vi "Actor Core.vi"(8 "error in":errorcluster caption="错误输入", 11 "Programmatic Controller in":refnum<class "Programmatic Controller.lvclass"> caption="操作者输入") -> (0 "error out":errorcluster caption="错误输出", 3 "Actor out":refnum<class "Actor.lvclass"> caption="操作者输出")   [LabVIEW 2017, in "Programmatic Controller.lvclass"]
doc: "(<B>Filename</B>: Actor Framework.lvlib:Actor.lvclass:Actor Core.vi)\n\nReceives messages to the actor, reacts to them, and initiates any error handling that may shut the actor down.\n\nDescendant classes may override this VI to append parallel tasks for the actor to complete while it handles messages. Overrides use the Call Parent Method node."
uses:
  Programmatic Controller.lvclass
  E:/Program Files (x86)/National Instruments/LabVIEW 2017/vi.lib/ActorFramework/Actor/Actor.lvclass
  <vilib>/ActorFramework/Actor/Actor.lvclass
  <vilib>/ActorFramework/Actor/Actor.lvclass/Actor.ctl
  <vilib>/ActorFramework/Message Enqueuer/Message Enqueuer.lvclass/Message Enqueuer.ctl
  <vilib>/Utility/error.llb/DialogType.ctl
  <vilib>/DAQmx/write.llb/DAQmx Write (Digital Bool 1Line 1Point).vi
  <vilib>/DAQmx/write.llb/DAQmx Write (Analog 1D DBL NChan 1Samp).vi
  <vilib>/ActorFramework/Message Enqueuer/Init from Existing Queue.vi
  <vilib>/ActorFramework/Message Enqueuer/Enqueue.vi
  <vilib>/ActorFramework/Stop Msg/Stop Msg.lvclass
  E:/Program Files (x86)/National Instruments/LabVIEW 2017/vi.lib/ActorFramework/Message/Message.lvclass
  <vilib>/ActorFramework/Message Priority Queue/Priority Enqueue.vi
  <vilib>/Utility/file.llb/Read Delimited Spreadsheet (DBL).vi
  <vilib>/DAQmx/create/channels.llb/DAQmx Create Channel (DO-Digital Output).vi
  <vilib>/DAQmx/create/channels.llb/DAQmx Create Channel (AO-Voltage-Basic).vi
  <vilib>/DAQmx/miscellaneous.llb/DAQmx Fill In Error Info.vi
  Printer Controller/Printer Controller/Printer Controller.lvclass
  <vilib>/ActorFramework/Message Enqueuer/Message Enqueuer.lvclass
panel:
  out "布尔 2":bool
  out "布尔":bool
  in  "打印开始":bool
  in  "lines":tag="Dev1/port0/line0" caption="线"
  out "G":dbl
  out "Z":dbl
  out "Y":dbl
  out "X":dbl
  in  "file path (dialog if empty)":path=path "C:/Users/whq/Documents/labview demo/TPP path demo/Matlab/save_test.txt" caption="文件路径 （空时为对话框）"
  in  "停止 2":bool
  in  "最大电压":dbl=10.0
  in  "最小电压":dbl=-10.0
  in  "物理通道":tag="Dev1/ao0:1"
  in  "停止":bool
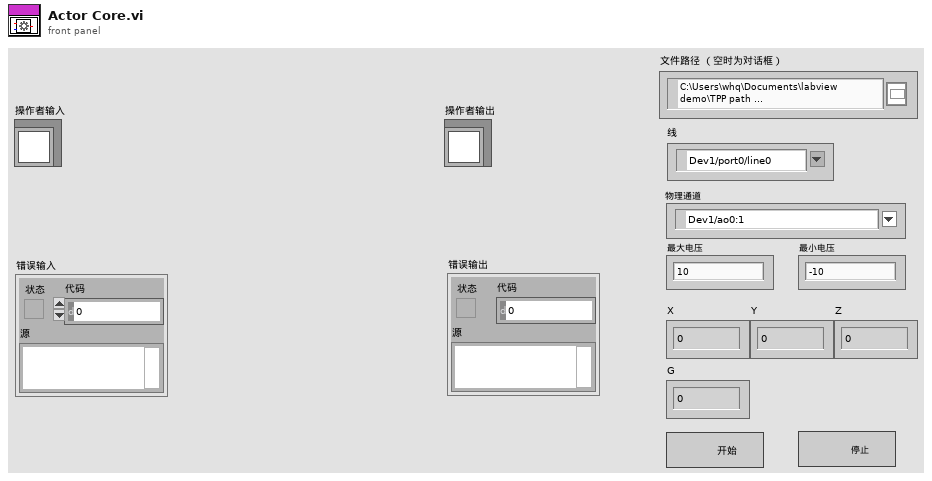
[diagram p1: front panel]
types:
  T1 = typedef "DialogType.ctl" = u16
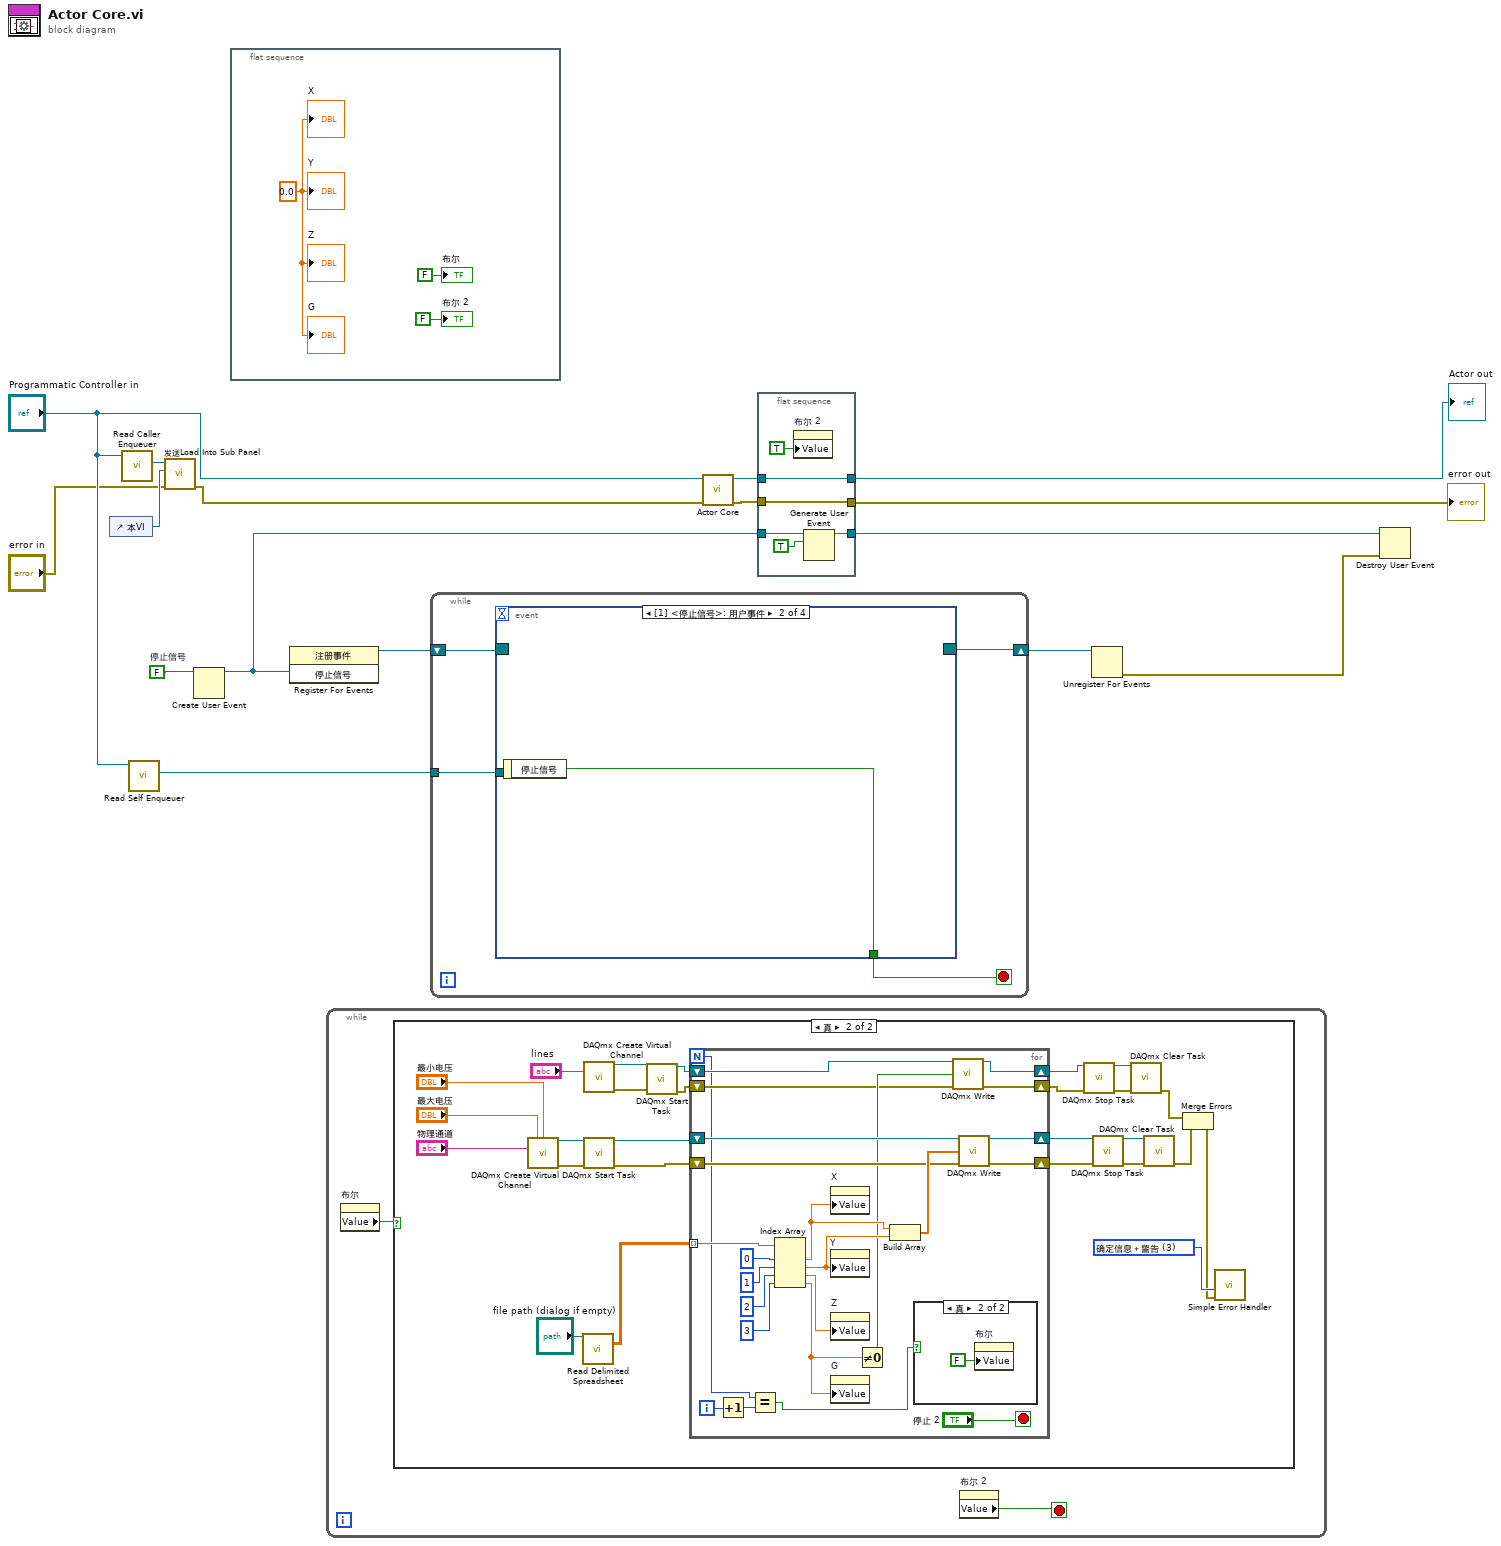
[diagram p0: block diagram]
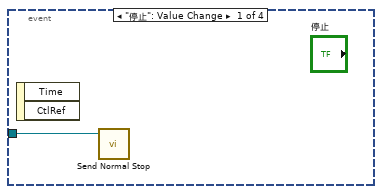
[diagram p4: hidden frame]
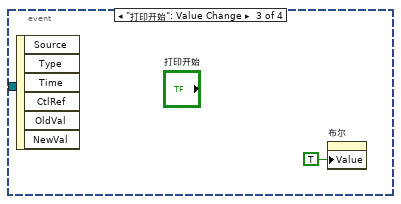
[diagram p5: hidden frame]
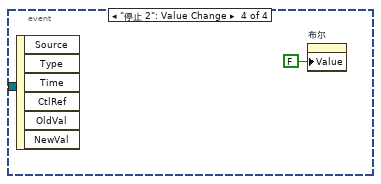
[diagram p6: hidden frame]
diagram:
  w14 = FALSE  # 停止信号
  n1 = control-ref of="本VI"() -> (w15:refnum<vi>)
  n2 = call <vilib>:"Read Caller Enqueuer.vi"("Actor"="Programmatic Controller in") -> ("Caller Enqueuer"=w16:refnum<class "Message Enqueuer.lvclass">)  [unwired: 10 in]
  n3 = call <vilib>:"Read Self Enqueuer.vi"("Actor"="Programmatic Controller in") -> ("Self Enqueuer"=w12:refnum<class "Message Enqueuer.lvclass">)  [unwired: 10 in]
  n4 = call "发送Load Into Sub Panel.vi"("error in (no error)"="error in", "VI引用"=w15, "Message Enqueuer"=w16) -> ("error out"=w9:errorcluster)  [unwired: 7 in, 1 out]
  n5 = Create User Event(user event datatype=w14) -> (user event=w8:refnum<user-event>)  [unwired: 1 in, 1 out]
  n6 = flat-sequence {
    frame #0 {
      w18 = 0.0 ("X")
      "X" <- w18
      "Y" <- w18
      "Z" <- w18
      "G" <- w18
      "布尔 2" <- FALSE ("布尔 2")
      "布尔" <- FALSE ("布尔")
    }
  }
  n7 = register-events(w8) -> (reference out=w13:refnum<event-registration>)  [unwired: 2 in, 1 out]
  n8 = while {
    stop <- w21 stop-if-true
    n9 = property on="布尔" class="Bool (严格)"() -> ("Value"=w20:bool)  [unwired: 2 in, 2 out]
    n10 = case shown="真" w20 {
      frame False {
      }
      frame True {
        w29 = T1 3 items=["无对话框", "确定信息", "继续或停止信息", "确定信息＋警告", "继续/停止＋警告"] ("对话框类型（确定信息：1）")
        n11 = call-poly <vilib>:"DAQmx Create Virtual Channel.vi"("maximum value"="最大电压", "minimum value"="最小电压", "physical channels"="物理通道") -> ("task out"=w39:refnum<k21>, "error out"=w40:errorcluster)  [unwired: 11 in]
        n12 = call-poly <vilib>:"Read Delimited Spreadsheet.vi"("file path (dialog if empty)"="file path (dialog if empty)") -> ("all rows"=w46:dbl[][])  [unwired: 9 in, 5 out]
        n13 = call-poly <vilib>:"DAQmx Create Virtual Channel.vi"("lines"="lines") -> ("task out"=w45:refnum<k21>, "error out"=w44:errorcluster)  [unwired: 13 in]
        n14 = call <vilib>:"DAQmx Start Task.vi"("task/channels in"=w39, "error in"=w40) -> ("task out"=w35:refnum<k21>, "error out"=w34:errorcluster)  [unwired: 12 in]
        n15 = call <vilib>:"DAQmx Start Task.vi"("task/channels in"=w45, "error in"=w44) -> ("task out"=w42:refnum<k21>, "error out"=w41:errorcluster)  [unwired: 12 in]
        n16 = for {
          N -> [w50]
          tunnel: w46 -> [w71] mode=indexing
          shift-right: [w69] -> w25
          shift-left: w34 -> [w60]
          shift-right: [w70] -> w26
          shift-left: w35 -> [w59]
          shift-right: [w53] -> w28
          shift-left: w41 -> [w56]
          shift-right: [w54] -> w27
          shift-left: w42 -> [w55]
          i -> [w52]
          stop <- "停止 2" stop-if-true
          n17 = Increment(x=w52) -> (x+1=w51:i32)
          n18 = Equal?(x=w50, y=w51) -> (x = y?=w49:bool)
          n19 = Index Array(array=w71, index #1=0 ("索引"), index #2=1 ("索引"), index #3=2 ("索引"), index #4=3 ("索引")) -> (element #1=w63:dbl, element #2=w62:dbl, element #3=w64:dbl, element #4=w58:dbl)
          n20 = property on="X" class="DigNum (严格)"("Value"=w63) -> ()  [unwired: 2 in, 2 out]
          n21 = property on="Y" class="DigNum (严格)"("Value"=w62) -> ()  [unwired: 2 in, 2 out]
          n22 = property on="Z" class="DigNum (严格)"("Value"=w64) -> ()  [unwired: 2 in, 2 out]
          n23 = property on="G" class="DigNum (严格)"("Value"=w58) -> ()  [unwired: 2 in, 2 out]
          n24 = Not Equal To 0?(x=w58) -> (x != 0?=w57:bool)
          n25 = Build Array(w63, w62) -> (w61:dbl[])
          n26 = case shown="真" w49 {
            frame False {
            }
            frame True {
              n27 = property on="布尔" class="Bool (严格)"("Value"=FALSE ("布尔")) -> ()  [unwired: 2 in, 2 out]
            }
          }
          n28 = call-poly <vilib>:"DAQmx Write.vi"("task/channels in"=w55, "data"=w57, "error in"=w56) -> ("task out"=w54:refnum<k21>, "error out"=w53:errorcluster)  [unwired: 10 in, 1 out]
          n29 = call-poly <vilib>:"DAQmx Write.vi"("task/channels in"=w59, "data"=w61, "error in"=w60) -> ("task out"=w70:refnum<k21>, "error out"=w69:errorcluster)  [unwired: 10 in, 1 out]
        }
        n30 = call <vilib>:"DAQmx Stop Task.vi"("task/channels in"=w27, "error in"=w28) -> ("task out"=w33:refnum<k21>, "error out"=w32:errorcluster)  [unwired: 12 in]
        n31 = call <vilib>:"DAQmx Stop Task.vi"("task/channels in"=w26, "error in"=w25) -> ("task out"=w30:refnum<k21>, "error out"=w31:errorcluster)  [unwired: 12 in]
        n32 = call <vilib>:"DAQmx Clear Task.vi"("task in"=w33, "error in"=w32) -> ("error out"=w24:errorcluster)  [unwired: 13 in]
        n33 = call <vilib>:"DAQmx Clear Task.vi"("task in"=w30, "error in"=w31) -> ("error out"=w23:errorcluster)  [unwired: 13 in]
        n34 = Merge Errors(w24, w23) -> (w22:errorcluster)
        n35 = call <vilib>:"Simple Error Handler.vi"("type of dialog (OK msg:1)"=w29, "error in (no error)"=w22) -> ()  [unwired: 3 in, 5 out]
      }
    }
    n36 = property on="布尔 2" class="Bool (严格)"() -> ("Value"=w21:bool)  [unwired: 2 in, 2 out]
  }
  n37 = while {
    shift-right: [w73] -> w5
    shift-left: w13 -> [w76]
    tunnel: w12 -> [w75]
    stop <- w74 stop-if-true
    n38 = event shown="[1] <停止信号>: 用户事件" {
      selector: w76 -> [_ _ _ _]
      dyn-events: [_ _ _ _] -> w73
      timeout: _ -> [_ _ _ _]
      tunnel: w75 -> [w77 _ _ _]
      tunnel: [_ w78 _ _] -> w74
      event "停止": Value Change {
        n39 = event-data() -> ()  [unwired: 1 in, 2 out]
        n40 = call <vilib>:"Send Normal Stop.vi"("Message Enqueuer"=w77) -> ()  [unwired: 10 in, 1 out]
      }
      event User Event {
        n41 = event-data() -> ("停止信号"=w78:bool)  [unwired: 1 in]
      }
      event "打印开始": Value Change {
        n42 = event-data() -> ()  [unwired: 1 in, 6 out]
        n43 = property on="布尔" class="Bool (严格)"("Value"=TRUE ("布尔")) -> ()  [unwired: 2 in, 2 out]
      }
      event "停止 2": Value Change {
        n44 = event-data() -> ()  [unwired: 1 in, 6 out]
        n45 = property on="布尔" class="Bool (严格)"("Value"=FALSE ("布尔")) -> ()  [unwired: 2 in, 2 out]
      }
    }
  }
  n46 = call-parent "Actor Core.vi"("error in"=w9, "Actor in"="Programmatic Controller in") -> ("error out"=w7:errorcluster, "Actor out"=w2:refnum<class "Actor.lvclass">)  [unwired: 8 in]
  n47 = flat-sequence {
    tunnel: w8 -> [w86]
    tunnel: w7 -> [w84]
    tunnel: [w84] -> w6
    tunnel: [w83] -> w3
    tunnel: [w82] -> w1
    tunnel: w2 -> [w82]
    frame #0 {
      n48 = property on="布尔 2" class="Bool (严格)"("Value"=TRUE ("布尔 2")) -> ()  [unwired: 2 in, 2 out]
      n49 = Generate User Event(user event=w86, event data cluster=TRUE ("事件数据")) -> (user event out=w83:refnum<user-event>)  [unwired: 2 in, 1 out]
    }
  }
  n50 = Unregister For Events(event registration refnum=w5) -> (error out=w4:errorcluster)  [unwired: 1 in]
  n51 = Destroy User Event(user event=w3, error in=w4) -> ()  [unwired: 1 out]
  "error out" <- w6
  "Actor out" <- w1
